vi "pop lower panel.vi"(1 "error in (no error)":errorcluster, 2 "Beamline Section":T1, 3 "pop vi":bool, 4 "Sub Panel":refnum<vi>) -> (0 "error out":errorcluster)   [LabVIEW 2016, in "main.lvlib"]
doc: "pop lower panel.vi \"pops\" out beamline section VI that is currently in lower sub-panel making it a stand-alone VI."
uses:
  main.lvlib
  main - slow.lvlib
  beamline selection.ctl
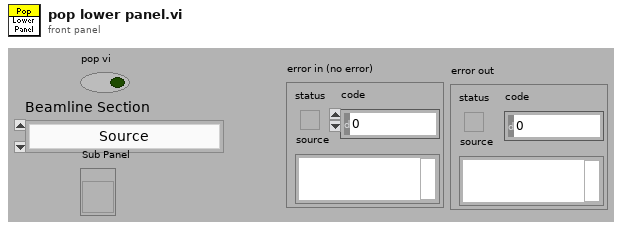
[diagram p1: front panel]
types:
  T1 = typedef "main.lvlib/beamline selection.ctl" = enum16{"Source", "Low End", "High End", "Transmission", "R30", "R45"}
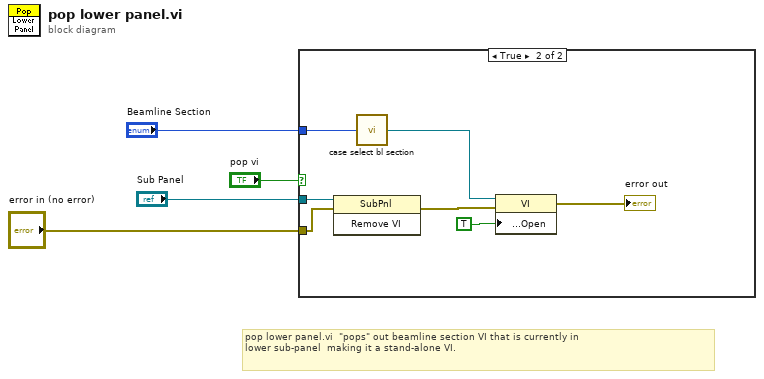
[diagram p0: block diagram]
diagram:
  # "pop lower panel.vi  \"pops\" out beamline section VI that is currently in \nlower sub-panel  making it a stand-alone VI."
  n1 = case shown="True" "pop vi" {
    tunnel: "Sub Panel" -> [_ w11]
    tunnel: "Beamline Section" -> [_ w8]
    tunnel: "error in (no error)" -> [_ w6]
    frame False {
    }
    frame True {
      n2 = invoke class="SubPnl" method="Remove VI"(reference=w11, error in=w6) -> (error out=w10:errorcluster)  [unwired: 1 in, 2 out]
      n3 = call "case select bl section.vi"("Beamline Section"=w8) -> ("VI Refnum"=w7:refnum<vi>)
      n4 = property class="VI"(reference=w7, error in=w10, "Front Panel.Open"=TRUE ("Front Panel Window:Open")) -> (error out=→"error out":errorcluster)  [unwired: 1 out]
    }
  }
